vi "Number of Permutations 2012 NIVerified.vi"(10 "R":i32, 11 "N":i32) -> (3 "Permutations":i32)   [LabVIEW 2019]
doc: "This VI calculates the number of permutations of a dataset based on its size and the size of the output you require."
uses:
  <vilib>/gmath/NI_Gmath.lvlib
panel:
  # "Overview: This VI  calculates the number of permutations of a dataset based on its size and the size of the output you require.\nRequirements: \nSoftware: LabVIEW 2012 (or compatible).\nInstructions: \n1. Specify the value of \"N\" and \"R\" for Permutations.\n2. Run the VI."
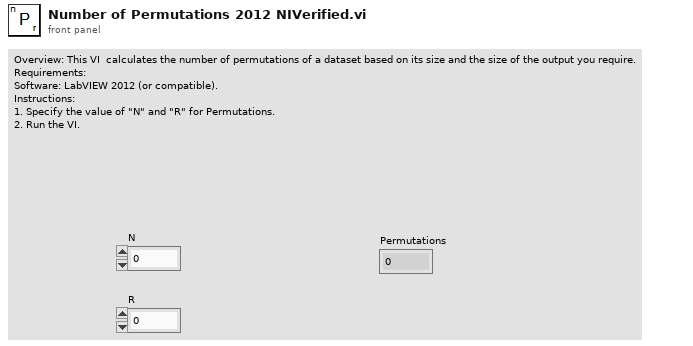
[diagram p1: front panel]
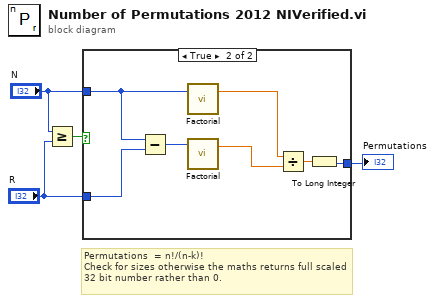
[diagram p0: block diagram]
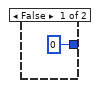
[diagram p2: hidden frame]
diagram:
  # "Permutations  = n!/(n-k)!\nCheck for sizes otherwise the maths returns full scaled 32 bit number rather than 0."
  n1 = Greater Or Equal?(x="N", y="R") -> (x >= y?=w3:bool)
  n2 = case shown="True" w3 {
    tunnel: "N" -> [_ w12]
    tunnel: "R" -> [_ w11]
    tunnel: [0 w7] -> w4
    frame False {
    }
    frame True {
      n3 = Subtract(x=w12, y=w11) -> (x-y=w10:i32)
      n4 = call <vilib>:"Factorial.vi"("n"=w12) -> ("n!"=w9:dbl)  [unwired: 2 in]
      n5 = call <vilib>:"Factorial.vi"("n"=w10) -> ("n!"=w6:dbl)  [unwired: 2 in]
      n6 = Divide(x=w9, y=w6) -> (x/y=w8:dbl)
      n7 = To Long Integer(number=w8) -> (32bit integer=w7:i32)
    }
  }
  "Permutations" <- w4
